vi "CRYNumber Format.vi"(8 "Notation":u16(slide), 9 "Digits":u16, 10 "Precision":u16(ring) items=["Digits of precision", "Significant digits"], 11 "Hide Trailing Zeros":bool caption="aa") -> (3 "Format string":string)   [LabVIEW 2013]
panel:
  in  "Num format":T1
  in  "Use Default":bool
  in  "Revert":bool
  in  "Cancel":bool
  in  "OK":bool
  out "Format":bool caption="aa"
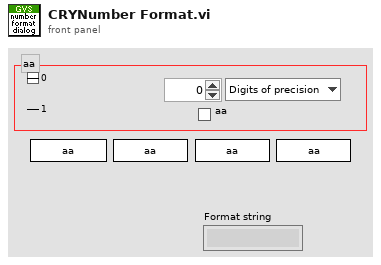
[diagram p1: front panel]
types:
  T1 = cluster{"Hide":string, "Precision":string, "Digits":string, "Notation":string}
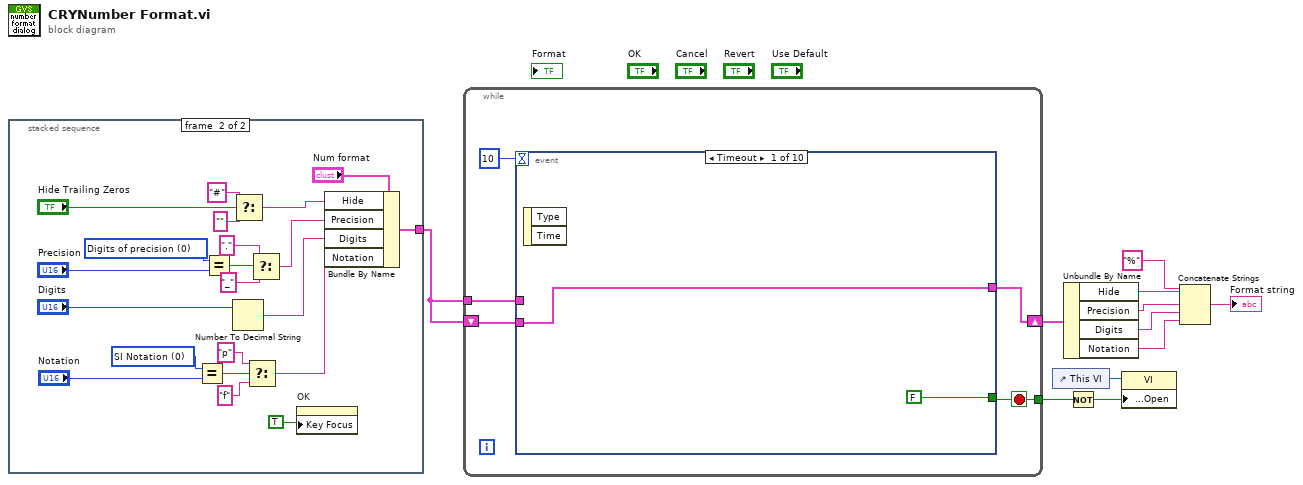
[diagram p0: block diagram]
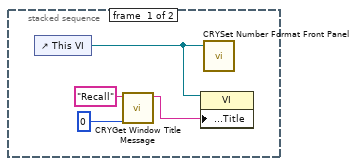
[diagram p2: hidden frame]
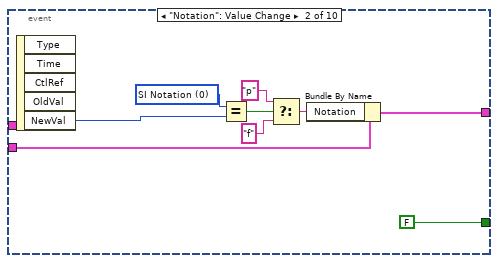
[diagram p3: hidden frame]
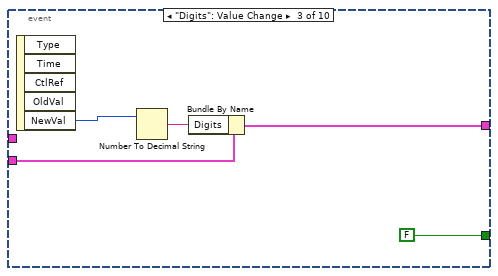
[diagram p4: hidden frame]
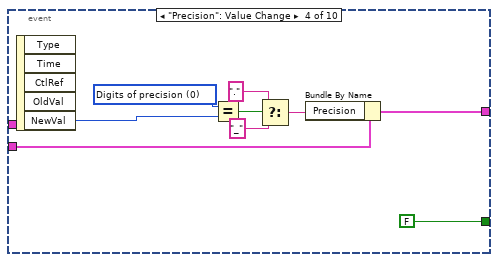
[diagram p5: hidden frame]
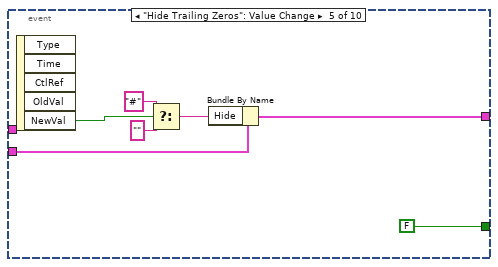
[diagram p6: hidden frame]
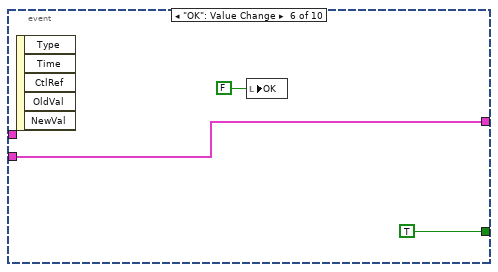
[diagram p7: hidden frame]
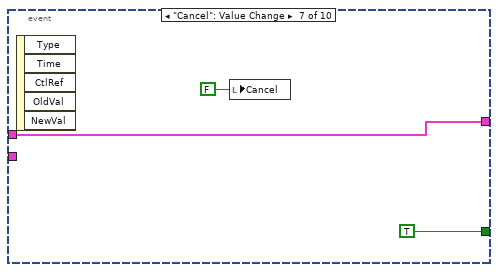
[diagram p8: hidden frame]
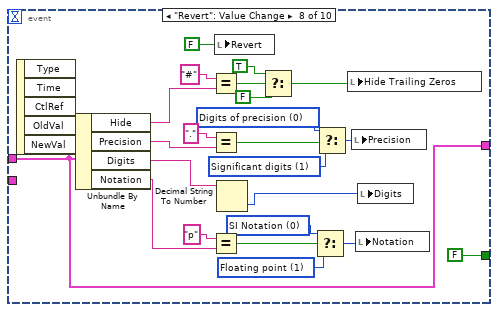
[diagram p9: hidden frame]
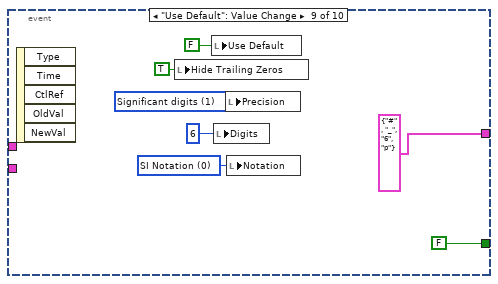
[diagram p10: hidden frame]
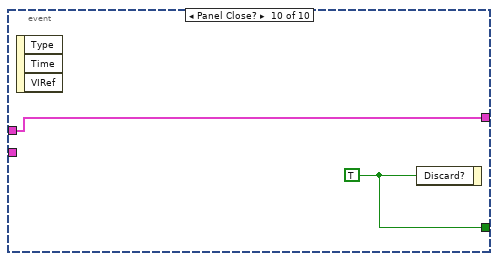
[diagram p11: hidden frame]
diagram:
  n1 = stacked-sequence {
    tunnel: [_ w17] -> w8
    frame #0 {
      n2 = control-ref of="This VI"() -> (w13:refnum<vi>)
      n3 = call "CRYGet Window Title Message.vi"("No"=0, "Kind"="Recall") -> ("Multibyte String"=w12:string)  [unwired: 4 in, 5 out]
      n4 = property class="VI"(reference=w13, "Front Panel.Title"=w12) -> ()  [unwired: 1 in, 2 out]
      n5 = call "CRYSet Number Format Front Panel.vi"("Vi Ref"=w13) -> ()  [unwired: 11 in]
    }
    frame #1 {
      w23 = u16 0 items=["SI Notation", "Floating point"] ("Notation")
      w28 = u16 0 items=["Digits of precision", "Significant digits"] ("Precision")
      n6 = Equal?(x=w23, y="Notation") -> (x = y?=w22:bool)
      n7 = Equal?(x=w28, y="Precision") -> (x = y?=w31:bool)
      n8 = Number To Decimal String(number="Digits") -> (decimal integer string=w24:string)  [unwired: 1 in]
      n9 = Select(t="#" ("format string"), s="Hide Trailing Zeros", f="" ("format string")) -> (s? t:f=w32:string)
      n10 = Select(t="p" ("string"), s=w22, f="f" ("string")) -> (s? t:f=w18:string)
      n11 = Select(t=".", s=w31, f="_") -> (s? t:f=w26:string)
      n12 = property on="OK" class="Bool (strict)"("Key Focus"=TRUE) -> ()  [unwired: 2 in, 2 out]
      n13 = Bundle By Name(cluster="Num format", "Hide"=w32, "Precision"=w26, "Digits"=w24, "Notation"=w18) -> (w17:T1)
    }
  }
  n14 = while {
    tunnel: [w40] -> w10
    shift-right: [w38] -> w7
    shift-left: w8 -> [w39]
    tunnel: w8 -> [w37]
    stop <- w40 stop-if-true
    n15 = event shown="[0] Timeout" {
      selector: _ -> [_ _ _ _ _ _ _ _ _ _]
      dyn-events: _ -> [_ _ _ _ _ _ _ _ _ _]
      timeout: 10 -> [_ _ _ _ _ _ _ _ _ _]
      tunnel: [FALSE ("Discard?") FALSE ("Discard?") FALSE ("Discard?") FALSE ("Discard?") FALSE ("Discard?") TRUE ("Discard?") TRUE ("Discard?") FALSE ("Discard?") FALSE ("Discard?") w111] -> w40
      tunnel: w39 -> [w42 w47 w55 w60 w70 w76 _ _ _ _]
      tunnel: [w42 w45 w54 w59 w68 w76 w78 w81 T1 {"Hide"="#", "Precision"="_", "Digits"="6", "Notation"="p"} ("Num format") w110] -> w38
      tunnel: w37 -> [_ _ _ _ _ _ w78 w81 _ w110]
      event Timeout {
        n16 = event-data() -> ()  [unwired: 1 in, 2 out]
      }
      event "Notation": Value Change {
        w49 = u16 0 items=["SI Notation", "Floating point"] ("Notation")
        n17 = event-data() -> ("NewVal"=w48:u16)  [unwired: 1 in, 4 out]
        n18 = Equal?(x=w49, y=w48) -> (x = y?=w50:bool)
        n19 = Select(t="p" ("string"), s=w50, f="f" ("string")) -> (s? t:f=w46:string)
        n20 = Bundle By Name(cluster=w47, "Notation"=w46) -> (w45:T1)
      }
      event "Digits": Value Change {
        n21 = event-data() -> ("NewVal"=w57:u16)  [unwired: 1 in, 4 out]
        n22 = Number To Decimal String(number=w57) -> (decimal integer string=w56:string)  [unwired: 1 in]
        n23 = Bundle By Name(cluster=w55, "Digits"=w56) -> (w54:T1)
      }
      event "Precision": Value Change {
        w63 = u16 0 items=["Digits of precision", "Significant digits"] ("Precision")
        n24 = event-data() -> ("NewVal"=w62:u16)  [unwired: 1 in, 4 out]
        n25 = Equal?(x=w63, y=w62) -> (x = y?=w64:bool)
        n26 = Select(t=".", s=w64, f="_") -> (s? t:f=w61:string)
        n27 = Bundle By Name(cluster=w60, "Precision"=w61) -> (w59:T1)
      }
      event "Hide Trailing Zeros": Value Change {
        n28 = event-data() -> ("NewVal"=w71:bool)  [unwired: 1 in, 4 out]
        n29 = Select(t="#" ("format string"), s=w71, f="" ("format string")) -> (s? t:f=w69:string)
        n30 = Bundle By Name(cluster=w70, "Hide"=w69) -> (w68:T1)
      }
      event "OK": Value Change {
        n31 = event-data() -> ()  [unwired: 1 in, 5 out]
        n32 = local write "OK"(FALSE ("OK")) -> ()
      }
      event "Cancel": Value Change {
        n33 = event-data() -> ()  [unwired: 1 in, 5 out]
        n34 = local write "Cancel"(FALSE ("Cancel")) -> ()
      }
      event "Revert": Value Change {
        w83 = u16 1 items=["SI Notation", "Floating point"] ("Notation")
        w84 = u16 0 items=["SI Notation", "Floating point"] ("Notation")
        w92 = u16 0 items=["Digits of precision", "Significant digits"] ("Precision")
        w91 = u16 1 items=["Digits of precision", "Significant digits"] ("Precision")
        n35 = event-data() -> ()  [unwired: 1 in, 5 out]
        n36 = Unbundle By Name(w81) -> ("Hide"=w101:string, "Precision"=w94:string, "Digits"=w89:string, "Notation"=w86:string)
        n37 = Equal?(x="#" ("format string"), y=w101) -> (x = y?=w99:bool)
        n38 = Equal?(x="." ("format string"), y=w94) -> (x = y?=w93:bool)
        n39 = Equal?(x="p" ("format string"), y=w86) -> (x = y?=w85:bool)
        n40 = local write "Revert"(FALSE ("Revert")) -> ()
        n41 = Decimal String To Number(string=w89) -> (number=w88:i32)  [unwired: 2 in, 1 out]
        n42 = Select(t=TRUE ("Revert"), s=w99, f=FALSE) -> (s? t:f=w96:bool)
        n43 = Select(t=w84, s=w85, f=w83) -> (s? t:f=w82:u16)
        n44 = Select(t=w92, s=w93, f=w91) -> (s? t:f=w90:u16)
        n45 = local write "Hide Trailing Zeros"(w96) -> ()
        n46 = local write "Precision"(w90) -> ()
        n47 = local write "Notation"(w82) -> ()
        n48 = local write "Digits"(w88) -> ()
      }
      event "Use Default": Value Change {
        w106 = u16 0 items=["SI Notation", "Floating point"] ("Notation")
        w108 = u16 1 items=["Digits of precision", "Significant digits"] ("Precision")
        n49 = event-data() -> ()  [unwired: 1 in, 5 out]
        n50 = local write "Hide Trailing Zeros"(TRUE ("Hide Traling Zeros")) -> ()
        n51 = local write "Use Default"(FALSE ("Use Default")) -> ()
        n52 = local write "Digits"(u16 6 ("Digits")) -> ()
        n53 = local write "Precision"(w108) -> ()
        n54 = local write "Notation"(w106) -> ()
      }
      event Panel Close? {
        w111 = TRUE ("Discard?")
        n55 = event-data() -> ()  [unwired: 1 in, 3 out]
        n56 = event-data("Discard?"=w111) -> ()  [unwired: 1 in, 1 out]
      }
    }
  }
  n57 = control-ref of="This VI"() -> (w11:refnum<vi>)
  n58 = Unbundle By Name(w7) -> ("Hide"=w5:string, "Precision"=w4:string, "Digits"=w3:string, "Notation"=w2:string)
  n59 = Not(x=w10) -> (.not. x?=w9:bool)
  n60 = property class="VI"(reference=w11, "Front Panel.Open"=w9) -> ()  [unwired: 1 in, 2 out]
  n61 = Concatenate Strings("%" ("string"), w5, w4, w3, w2) -> (→"Format string":string)
